vi "GetMonthlyComics.vi"(8 "error in":errorcluster) -> (0 "error out":errorcluster)   [LabVIEW 2024]
uses:
  <vilib>/addons/_JKI.lib/REST Client/classes/REST Client/REST Client.lvclass
panel:
  in  "Stop":bool
  out "last offset":i32
  out "progress":i32(slide) caption="60 of 73" scale=0.0..73.0
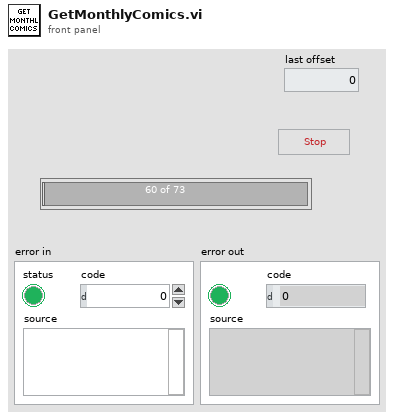
[diagram p1: front panel]
types:
  T1 = typedef "comics.reply--cluster.ctl" = cluster{"code":i32, "status":string, "etag":string, "data":cluster{"offset":i32, "limit":i32, "total":i32, "count":i32, "results":T2[]}}
  T2 = typedef "comic--cluster.ctl" = cluster{"id":i32, "digitalId":i32, "title":string, "issueNumber":i32, "variantDescription":string, "description":string, "modified":variant, "upc":string, "format":string, "pageCount":i32, "resourceURI":string, "urls":cluster{"type":string, "url":string}[], "series":cluster{"resourceURI":string, "name":string}, "dates":cluster{"type":string, "date":string}[], "prices":cluster{"price":dbl, "type":string}[], "thumbnail":cluster{"path":string, "extension":string}, "images":cluster{"path":string, "extension":string}[], "creators":cluster{"available":i32, "returned":i32, "collectionURI":string, "items":cluster{"resourceURI":string, "name":string, "role":string}[]}, "characters":cluster{"available":i32, "returned":i32, "collectionURI":string, "items":cluster{"resourceURI":string, "name":string}[]}, "stories":cluster{"available":i32, "returned":i32, "collectionURI":string, "items":cluster{"resourceURI":string, "name":string, "type":string}[]}, "events":cluster{"available":i32, "returned":i32, "collectionURI":string, "items":cluster{"resourceURI":string, "name":string}[]}}
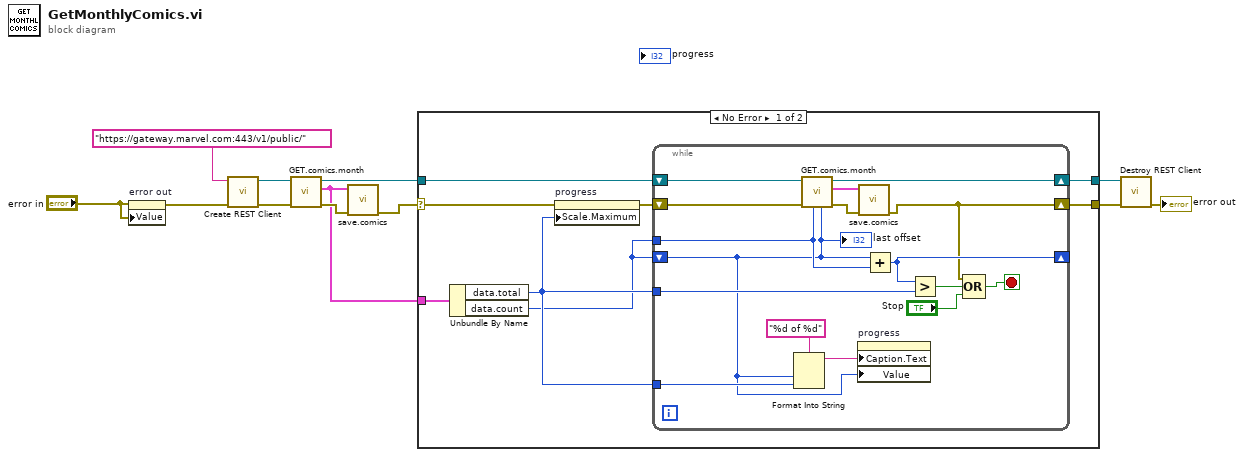
[diagram p0: block diagram]
diagram:
  n1 = property on="error out" class="Clust (strict)"(error in="error in", "Value"="error in") -> (error out=w2:errorcluster)  [unwired: 1 in, 1 out]
  n2 = call <vilib>:"Create REST Client.vi"("error in (no error)"=w2, "Base URL"="https://gateway.marvel.com:443/v1/public/") -> ("error out"=w10:errorcluster, "REST Client out"=w11:refnum<class "REST Client.lvclass">)  [unwired: 8 in]
  n3 = call "GET.comics.month.vi"("error in (no error)"=w10, "REST Client in"=w11) -> ("error out"=w8:errorcluster, "data"=w7:T1, "REST Client out"=w6:refnum<class "REST Client.lvclass">)  [unwired: 7 in]
  n4 = call "save.comics.vi"("error in"=w8, "data"=w7) -> ("error out"=w3:errorcluster)  [unwired: 9 in]
  n5 = case shown="No Error" w3 {
    selector: w3 -> [w14 w37]
    tunnel: w7 -> [w20 _]
    tunnel: w6 -> [w19 w38]
    tunnel: [w18 w38] -> w5
    tunnel: [w17 w37] -> w4
    frame No Error {
      n6 = Unbundle By Name(w20) -> ("data.total"=w15:i32, "data.count"=w13:i32)
      n7 = property on="progress" class="Slide (strict)"(error in=w14, "Scale.Maximum"=w15) -> (error out=w16:errorcluster)  [unwired: 1 in, 1 out]
      n8 = while {
        shift-right: [w33] -> w18
        shift-left: w19 -> [w34]
        shift-right: [w27] -> w17
        shift-left: w16 -> [w32]
        tunnel: w13 -> [w31]
        shift-right: [w30] -> _
        shift-left: w13 -> [w22]
        tunnel: w15 -> [w29]
        tunnel: w15 -> [w24]
        stop <- w26 stop-if-true
        n9 = Format Into String(format string="%d of %d", w22, w24) -> (resulting string=w23:string)  [unwired: 2 in, 1 out]
        n10 = call "GET.comics.month.vi"("series offset"=w22, "Number of Series to GET"=w31, "error in (no error)"=w32, "REST Client in"=w34) -> ("error out"=w35:errorcluster, "data"=w36:T1, "REST Client out"=w33:refnum<class "REST Client.lvclass">)  [unwired: 5 in]
        n11 = property on="progress" class="Slide (strict)"("Caption.Text"=w23, "Value"=w22) -> ()  [unwired: 2 in, 2 out]
        n12 = call "save.comics.vi"("error in"=w35, "data"=w36) -> ("error out"=w27:errorcluster)  [unwired: 9 in]
        n13 = Add(x=w22, y=w31) -> (x+y=w30:i32)
        n14 = Greater?(x=w30, y=w29) -> (0:w28:bool)
        n15 = Compound Arithmetic op=OR(w27, w28, "Stop") -> (w26:bool)
        "last offset" <- w22
      }
    }
    frame Error {
    }
  }
  n16 = call-dynamic "Destroy REST Client.vi"("error in (no error)"=w4, "REST Client in"=w5) -> ("error out"=→"error out":errorcluster)  [unwired: 9 in]
